vi "Add Report Section.vi"(6 "Step Number":i32, 7 "Report Path":path, 8 "error in (no error)":errorcluster, 9 "Result":T1, 10 "Report in":refnum<class "NI_report.lvclass">, 11 "Step in":refnum<class "Step.lvclass">) -> (0 "error out":errorcluster, 2 "Report out":refnum<class "NI_report.lvclass">, 3 "Step out":refnum<class "Step.lvclass">)   [LabVIEW 2020, in "MacroAssert.lvlib" / "Step.lvclass"]
uses:
  Step.lvclass
  <vilib>/Utility/NIReport.llb/NI_report.lvclass
  CTLs/Result.ctl
  CTLs/Outcome.ctl
  <vilib>/Utility/NIReport.llb/Append Report Text (str wrap).vi
  MacroAssert.lvlib
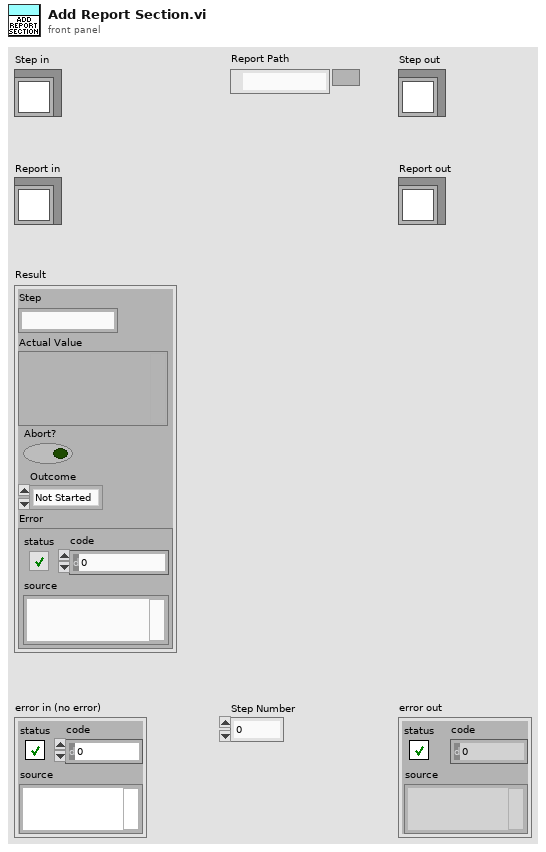
[diagram p1: front panel]
types:
  T1 = typedef "MacroAssert.lvlib/Result.ctl" = cluster{"Step":string, "Actual Value":variant, "Abort?":bool, "Outcome":T2, "Error":errorcluster}
  T2 = typedef "MacroAssert.lvlib/Outcome.ctl" = enum16{"Not Started", "Skipped", "Pass", "Fail", "Complete", "Error", "Auto Abort", "User Abort"}
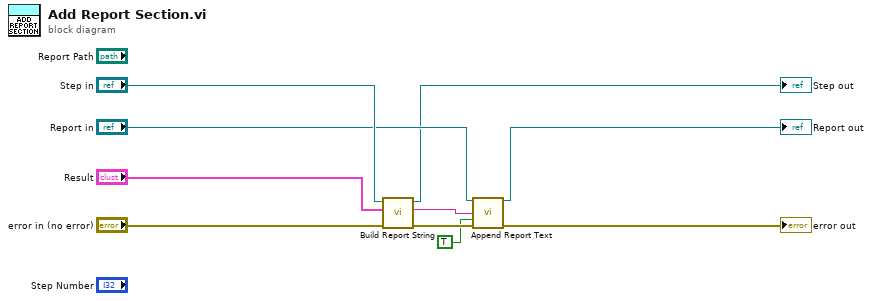
[diagram p0: block diagram]
diagram:
  n1 = call-dynamic "Build Report String.vi"("error in (no error)"="error in (no error)", "Result"="Result", "Step in"="Step in") -> ("error out"=w10:errorcluster, "Report String"=w1:string, "Step out"=→"Step out":refnum<class "Step.lvclass">)  [unwired: 6 in]
  n2 = call-poly <vilib>:"Append Report Text.vi"("report in"="Report in", "text"=w1, "append on new line? (F)"=TRUE, "error in (no error)"=w10) -> ("report out"=→"Report out":refnum<class "NI_report.lvclass">, "error out"=→"error out":errorcluster)  [unwired: 8 in, 2 out]
